vi "Convert Database Data to List.vi"(8 "error in (no error)":errorcluster, 10 "FetchedData":variant[](array[variant]), 11 "QDFunction in":refnum<class "QDList.lvclass">) -> (0 "error out":errorcluster, 1 "QDFunction Acronym":string, 2 "QDFunction Name":string, 3 "QDFunction out":refnum<class "QDList.lvclass">)   [LabVIEW 2015, in "QDList.lvclass"]
uses:
  QDList.lvclass
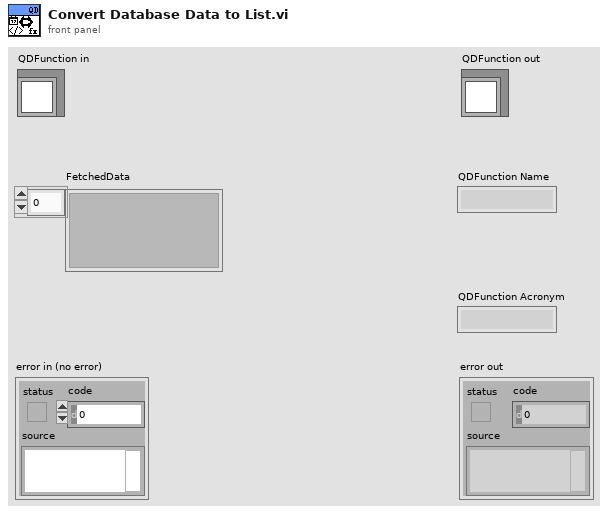
[diagram p1: front panel]
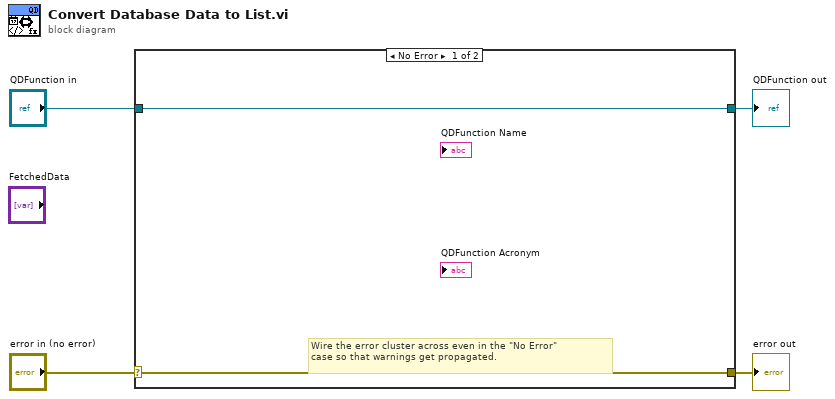
[diagram p0: block diagram]
diagram:
  n1 = case shown="No Error" "error in (no error)" {
    selector: "error in (no error)" -> [w5 w8]
    tunnel: [w5 w8] -> w3
    tunnel: [w6 w7] -> w1
    tunnel: "QDFunction in" -> [w6 w7]
    frame No Error {
      # "Wire the error cluster across even in the \"No Error\"\ncase so that warnings get propagated."
    }
    frame Error {
    }
  }
  "error out" <- w3
  "QDFunction out" <- w1
